vi "GetContentType.vi"(1 "ForceValue":string, 2 "File Path":path) -> (0 "Content Type":string)   [LabVIEW 2014]
doc: "Based on ending of File Path, choose appropriate Content Type.\nNote: enter values in \"ForceValue\" to ignore File Path and process Content Type using that instead. Leave Force Value blank (string of length zero) to operate on File Path normally."
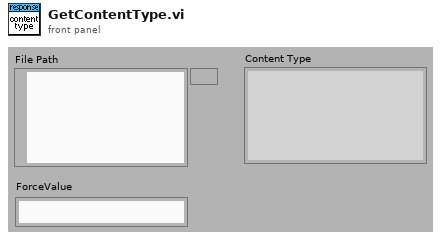
[diagram p1: front panel]
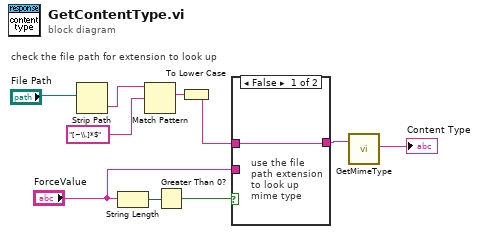
[diagram p0: block diagram]
diagram:
  # "check the file path for extension to look up"
  n1 = Strip Path(path="File Path") -> (name=w9:string)  [unwired: 1 out]
  n2 = String Length(string="ForceValue") -> (length=w6:i32)
  n3 = Match Pattern(string=w9, regular expression="[~\\.]*$") -> (match substring=w7:string)  [unwired: 4 out]
  n4 = Greater Than 0?(x=w6) -> (x > 0?=w5:bool)
  n5 = To Lower Case(string=w7) -> (all lower case string=w3:string)
  n6 = case shown="False" w5 {
    tunnel: "ForceValue" -> [_ w12]
    tunnel: [w11 w12] -> w2
    tunnel: w3 -> [w11 _]
    frame False {
      # "use the file\npath extension\nto look up\nmime type"
    }
    frame True {
      # "use the\nforce value"
    }
  }
  n7 = call <userlib>:"GetMimeType.vi"("Extension"=w2) -> ("mimetype"=→"Content Type":string)  [unwired: 2 in]
